vi "ReadRadsensoren.vi"(8 "error in (no error)":errorcluster, 9 "milliseconds to wait":u32, 10 "FPGA VI Reference Out":refnum<k20>) -> (0 "error out":errorcluster)   [LabVIEW 2016]
uses:
  <vilib>/Utility/error.llb/Error Cluster From Error Code.vi
  <vilib>/rvi/errors/niLvFpgaAdjustHostInterfaceError.vi
  Globale Variablen VI/RadSensoren.vi
  <vilib>/rvi/interface/nirviReadWriteControl/nirviReadWriteControl.xnode
  NiFpgaLv.dll
  <vilib>/rvi/interface/Simulation/niFpgaSimulationCallBeginRW.vi
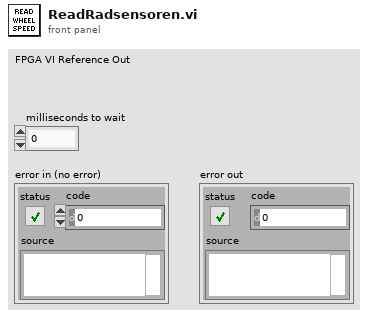
[diagram p1: front panel]
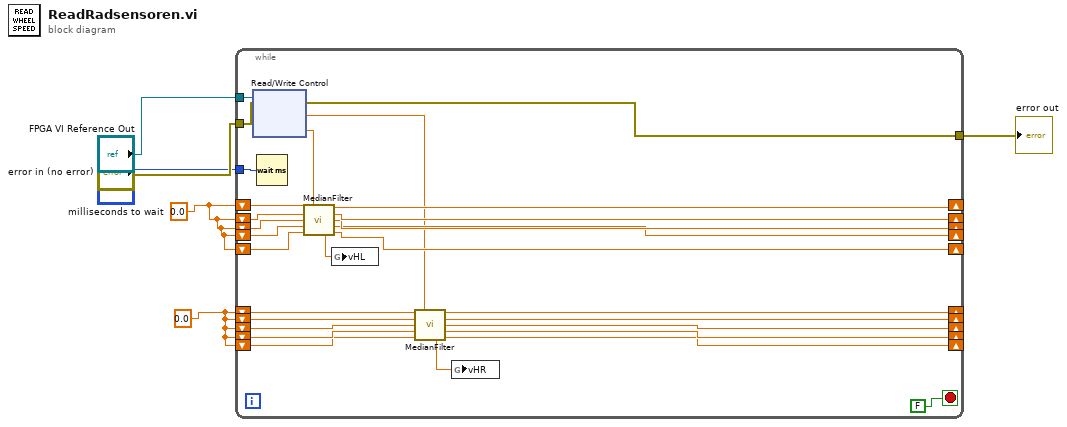
[diagram p0: block diagram]
diagram:
  w1 = 0.0
  w2 = 0.0
  n1 = while {
    tunnel: "error in (no error)" -> [w32]
    tunnel: [w31] -> w6
    tunnel: "milliseconds to wait" -> [w34]
    tunnel: "FPGA VI Reference Out" -> [w33]
    shift-right: [w23] -> _
    shift-left: w2 -> [w28]
    shift-right: [w22] -> _
    shift-left: w2 -> [w27]
    shift-right: [w21] -> _
    shift-left: w2 -> [w26]
    shift-right: [w20] -> _
    shift-left: w2 -> [w25]
    shift-right: [w19] -> _
    shift-left: w2 -> [w24]
    shift-right: [w16] -> _
    shift-left: w1 -> [w15]
    shift-right: [w14] -> _
    shift-left: w1 -> [w13]
    shift-right: [w12] -> _
    shift-left: w1 -> [w11]
    shift-right: [w10] -> _
    shift-left: w1 -> [w9]
    shift-right: [w8] -> _
    shift-left: w1 -> [w7]
    stop <- FALSE stop-if-true
    n2 = xnode "Read/Write Control"("FPGA VI Reference In"=w33, "error in"=w32) -> ("error out"=w31:errorcluster, "vHR"=w18:sgl, "vHL"=w30:sgl)  [unwired: 1 out]
    n3 = Wait (ms)(milliseconds to wait=w34) -> ()  [unwired: 1 out]
    n4 = call "MedianFilter.vi"("Numeric 9"=w28, "vHL"=w30, "Numeric 7"=w27, "Numeric 5"=w26, "Numeric 3"=w25, "Numeric in"=w24) -> ("Numeric 10"=w23:dbl, "Numeric 8"=w22:dbl, "Numeric 6"=w21:dbl, "Numeric 4"=w20:dbl, "OUTPUT"=w29:dbl, "Numeric 2"=w19:dbl)  [unwired: 4 in]
    n5 = global write "RadSensoren.vi" "vHL"(w29) -> ()
    n6 = call "MedianFilter.vi"("Numeric 9"=w15, "vHL"=w18, "Numeric 7"=w13, "Numeric 5"=w11, "Numeric 3"=w9, "Numeric in"=w7) -> ("Numeric 10"=w16:dbl, "Numeric 8"=w14:dbl, "Numeric 6"=w12:dbl, "Numeric 4"=w10:dbl, "OUTPUT"=w17:dbl, "Numeric 2"=w8:dbl)  [unwired: 4 in]
    n7 = global write "RadSensoren.vi" "vHR"(w17) -> ()
  }
  "error out" <- w6
